vi "DB_InsertData.vi"(8 "error in (no error)":errorcluster, 9 "Entry Console":T1, 10 "ID":string, 11 "SQLite Connection in":refnum<class "Connection.lvclass">) -> (0 "error out":errorcluster, 3 "SQLite Connection":refnum<class "Connection.lvclass">)   [LabVIEW 2020]
doc: "Inserts car ID and washing options into to the database."
uses:
  <vilib>/drjdpowell/SQLite Library/SQL Connection/Connection.lvclass
  <vilib>/drjdpowell/SQLite Library/SQL Statement/SQL Statement.lvclass/SQL Statement.ctl
  <vilib>/drjdpowell/SQLite Library/SQL Statement/Bind Text.vi
  <vilib>/drjdpowell/SQLite Library/SQL Statement/Bind Integer.vi
  <vilib>/drjdpowell/SQLite Library/SQL Statement/Bind Timestamp (Real).vi
  <vilib>/drjdpowell/SQLite Library/SQL Statement/Step.vi
  <vilib>/drjdpowell/SQLite Library/SQL Statement/Bind Real.vi
  <vilib>/drjdpowell/SQLite Library/SQL Statement/Error Message.vi
  <vilib>/drjdpowell/SQLite Library/SQL Statement/Bind Parameters.vi
  <vilib>/drjdpowell/SQLite Library/SQL Statement/SQL Statement.lvclass
  <vilib>/drjdpowell/SQLite Library/Transaction Helpers/Transaction.lvlib
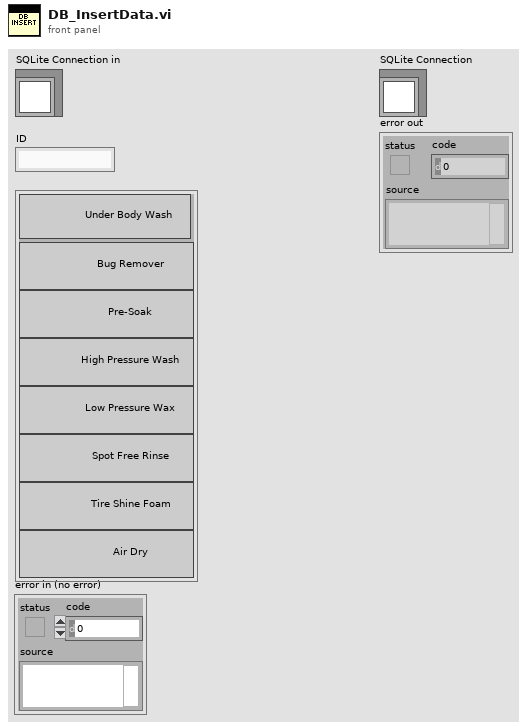
[diagram p1: front panel]
types:
  T1 = cluster{"Under Body Wash Button":bool, "Bug Remover Button":bool, "Pre-Soak Button":bool, "High Pressure Wash Button":bool, "Low Pressure Wax Button":bool, "Spot Free Rinse Button":bool, "Tire Shine Foam Button":bool, "Air Dry Button":bool}
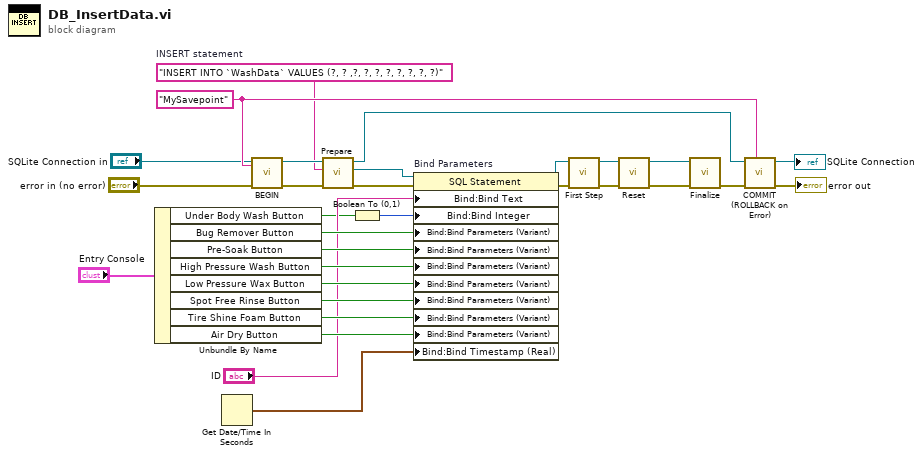
[diagram p0: block diagram]
diagram:
  w28 = "MySavepoint" ("Savepoint name")
  w23 = "INSERT INTO `WashData` VALUES (?, ? ,?, ?, ?, ?, ?, ?, ?, ?)"  # INSERT statement
  n1 = Unbundle By Name("Entry Console") -> ("Under Body Wash Button"=w2:bool, "Bug Remover Button"=w10:bool, "Pre-Soak Button"=w9:bool, "High Pressure Wash Button"=w8:bool, "Low Pressure Wax Button"=w7:bool, "Spot Free Rinse Button"=w6:bool, "Tire Shine Foam Button"=w5:bool, "Air Dry Button"=w4:bool)
  n2 = Get Date/Time In Seconds() -> (seconds since 1Jan1904=w12:timestamp)
  n3 = call <vilib>:"BEGIN.vi"("Savepoint name"=w28, "error in (no error)"="error in (no error)", "SQLite Connection in"="SQLite Connection in") -> ("error out"=w27:errorcluster, "SQLite Connection"=w26:refnum<class "Connection.lvclass">)  [unwired: 7 in]
  n4 = call <vilib>:"Prepare.vi"("error in (no error)"=w27, "SQL"=w23, "SQLite Connection in"=w26) -> ("error out"=w22:errorcluster, "SQL Statement"=w21:refnum<class "SQL Statement.lvclass">, "SQLite Connection"=w29:refnum<class "Connection.lvclass">)  [unwired: 4 in, 2 out]
  n5 = Boolean To (0,1)(Boolean=w2) -> (0, 1=w1:i16)
  n6 = property on="Bind Parameters" class="SQL Statement"(reference=w21, error in=w22, "Bind:Bind Text"="ID", "Bind:Bind Integer"=w1, "Bind:Bind Parameters (Variant)"=w10, "Bind:Bind Parameters (Variant)"=w9, "Bind:Bind Parameters (Variant)"=w8, "Bind:Bind Parameters (Variant)"=w7, "Bind:Bind Parameters (Variant)"=w6, "Bind:Bind Parameters (Variant)"=w5, "Bind:Bind Parameters (Variant)"=w4, "Bind:Bind Timestamp (Real)"=w12) -> (reference out=w20:refnum<class "SQL Statement.lvclass">, error out=w19:errorcluster)
  n7 = call <vilib>:"First Step.vi"("error in (no error)"=w19, "SQL Statement in"=w20) -> ("error out"=w18:errorcluster, "SQL Statement"=w17:refnum<class "SQL Statement.lvclass">)  [unwired: 7 in, 1 out]
  n8 = call <vilib>:"Reset.vi"("error in (no error)"=w18, "SQL Statement in"=w17) -> ("error out"=w25:errorcluster, "SQL Statement"=w24:refnum<class "SQL Statement.lvclass">)  [unwired: 8 in]
  n9 = call <vilib>:"Finalize.vi"("error in (no error)"=w25, "SQL Statement in"=w24) -> ("error out"=w30:errorcluster)  [unwired: 9 in]
  n10 = call <vilib>:"COMMIT (ROLLBACK on Error).vi"("Savepoint name"=w28, "error in (no error)"=w30, "SQLite Connection in"=w29) -> ("error out"=→"error out":errorcluster, "SQLite Connection"=→"SQLite Connection":refnum<class "Connection.lvclass">)  [unwired: 7 in]
